vi "LogMovementSteps.vi"(11 "Control Cluster":T1 {"Yaw Speed" scale=-1.0..1.0; "Vertical Speed" scale=-1.0..1.0; "Pitch" scale=-1.0..1.0; "Roll" scale=-1.0..1.0}) -> (0 "s? t:f 2":dbl, 3 "s? t:f":dbl)   [LabVIEW 2017]
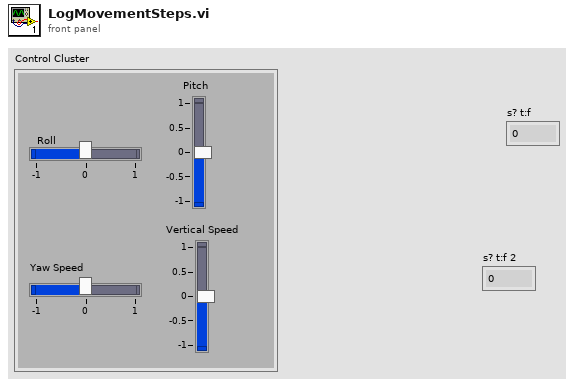
[diagram p1: front panel]
types:
  T1 = cluster{"Roll":sgl, "Pitch":sgl, "Vertical Speed":sgl, "Yaw Speed":sgl}
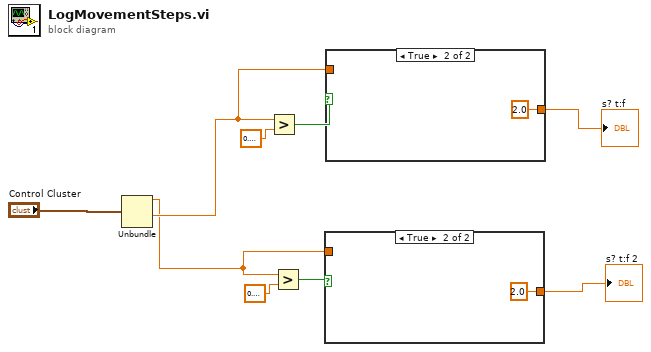
[diagram p0: block diagram]
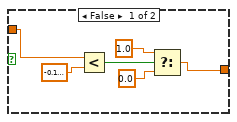
[diagram p2: hidden frame]
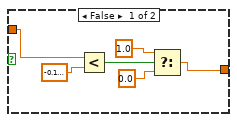
[diagram p3: hidden frame]
diagram:
  n1 = Unbundle("Control Cluster") -> ("Roll"=w1:sgl, "Vertical Speed"=w6:sgl)  [unwired: 2 out]
  n2 = Greater?(x=w6, y=sgl 0.1) -> (0:w7:bool)
  n3 = Greater?(x=w1, y=sgl 0.1) -> (0:w3:bool)
  n4 = case shown="True" w3 {
    tunnel: w1 -> [w15 _]
    tunnel: [w10 2.0 ("f")] -> w2
    frame False {
      n5 = Less?(x=w15, y=sgl -0.1) -> (x < y?=w13:bool)
      n6 = Select(t=1.0, s=w13, f=0.0) -> (s? t:f=w10:dbl)
    }
    frame True {
    }
  }
  "s? t:f 2" <- w2
  n7 = case shown="True" w7 {
    tunnel: w6 -> [w22 _]
    tunnel: [w17 2.0 ("f")] -> w5
    frame False {
      n8 = Less?(x=w22, y=sgl -0.1) -> (x < y?=w20:bool)
      n9 = Select(t=1.0, s=w20, f=0.0) -> (s? t:f=w17:dbl)
    }
    frame True {
    }
  }
  "s? t:f" <- w5
